vi "Build the ppl.vi"(8 "error in (no error)":errorcluster, 10 "Name of target (My Computer)":string="My Computer", 11 "Path override":path) -> (0 "error out":errorcluster, 3 "Generated files":path[](array[path]))   [LabVIEW 2021]
uses:
  <vilib>/AppBuilder/AB_API_Simple/Build (path).vi
  <vilib>/AppBuilder/AB_API_Simple/NI_App_Builder_API.lvlib
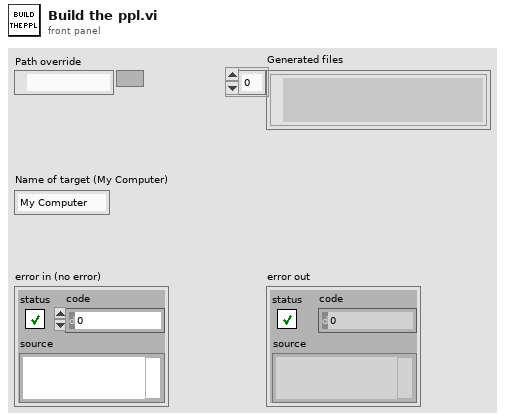
[diagram p1: front panel]
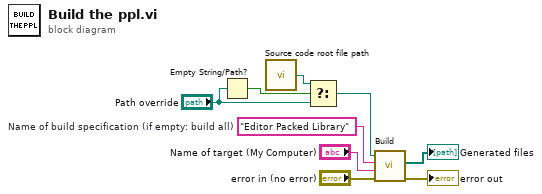
[diagram p0: block diagram]
diagram:
  w9 = "Editor Packed Library"  # Name of build specification (if empty: build all)
  n1 = Empty String/Path?(string/path="Path override") -> (empty?=w8:bool)
  n2 = call "Source code root file path.vi"() -> ("Source code root path"=w7:path)  [unwired: 1 in]
  n3 = Select(t=w7, s=w8, f="Path override") -> (s? t:f=w5:path)
  n4 = call-poly <vilib>:"Build.vi"("error in (no error)"="error in (no error)", "Name of target (My Computer)"="Name of target (My Computer)", "Name of build specification (if empty: build all)"=w9, "Path to project"=w5) -> ("error out"=→"error out":errorcluster, "Generated files"=→"Generated files":path[])  [unwired: 6 in]
